vi "Write Current.vi"(8 "error in":errorcluster, 10 "Current":dbl, 11 "6700C in":refnum<class "6700C.lvclass">) -> (0 "error out":errorcluster, 3 "6700C out":refnum<class "6700C.lvclass">)   [LabVIEW 2019, in "6700C.lvlib" / "6700C.lvclass"]
uses:
  Library/6700C.lvclass
  builds/Instruments/PowerSupply.lvlibp/Library/PowerSupply.lvclass
  builds/Engine/Engine.lvlibp/Project/Engine.lvclass
  C:/Users/Public/Documents/Development/builds/Engine/Engine.lvlibp/Project/Engine.lvclass
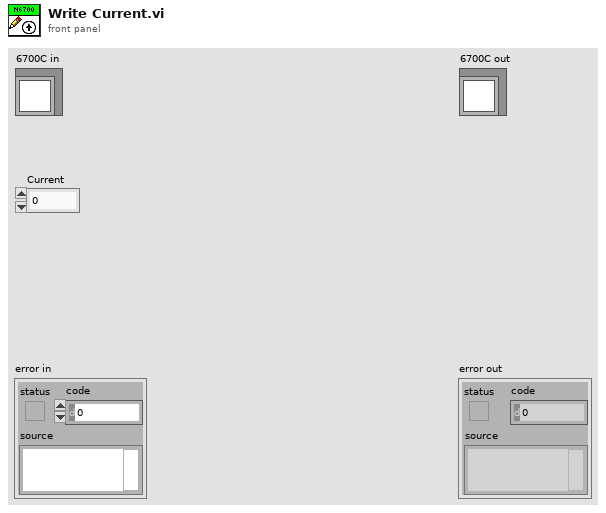
[diagram p1: front panel]
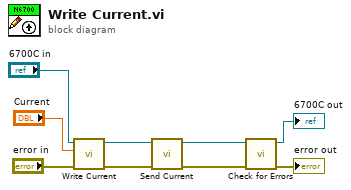
[diagram p0: block diagram]
diagram:
  n1 = call-parent "Write Current.vi"("error in"="error in", "Current"="Current", "PowerSupply in"="6700C in") -> ("error out"=w4:errorcluster, "PowerSupply out"=w3:refnum<class "6700C.lvclass">)  [unwired: 7 in]
  n2 = call "Send Current.vi"("error in"=w4, "6700C in"=w3) -> ("error out"=w1:errorcluster, "6700C out"=w2:refnum<class "6700C.lvclass">)  [unwired: 8 in]
  n3 = call "Check for Errors.vi"("error in"=w1, "Engine in"=w2) -> ("error out"=→"error out":errorcluster, "Engine out"=→"6700C out":refnum<class "6700C.lvclass">)  [unwired: 8 in]
